vi "subterm.vi"(1 "Escala":bool) -> (0 "Temperatura":dbl(slide) scale=0.0..212.0)   [LabVIEW 2017]
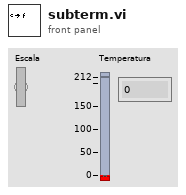
[diagram p1: front panel]
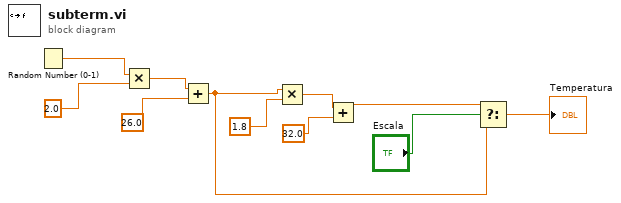
[diagram p0: block diagram]
diagram:
  n1 = Random Number (0-1)() -> (number: 0 to 1=w1:dbl)
  n2 = Multiply(x=w1, y=2.0) -> (x*y=w4:dbl)
  n3 = Add(x=w4, y=26.0) -> (x+y=w11:dbl)
  n4 = Multiply(x=w11, y=1.8) -> (x*y=w8:dbl)
  n5 = Add(x=w8, y=32.0) -> (x+y=w9:dbl)
  n6 = Select(t=w9, s="Escala", f=w11) -> (s? t:f=→"Temperatura":dbl)
